vi "tcs shm issue Command stop Motion LV.vi"(8 "error in (no error)":errorcluster, 11 "command_stopMotion_Ctl":cluster{"stopMotion":u8}) -> (0 "error out":errorcluster, 2 "function return":i32, 3 "command_stopMotion_Ctl out":cluster{"stopMotion":u8})   [LabVIEW 2016, in "SALLV_tcs.lvlib"]
doc: "int tcs_shm_issueCommand_stopMotionLV(tcs_command_stopMotionLV *command_stopMotion_Ctl );"
uses:
  SALLV_tcs.lvlib
  SALLV_tcs.so
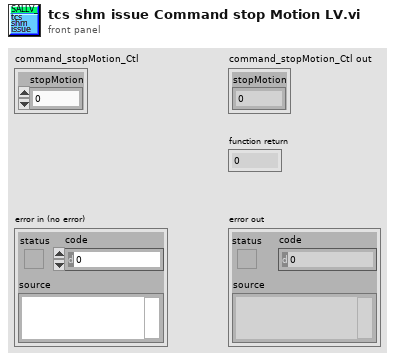
[diagram p1: front panel]
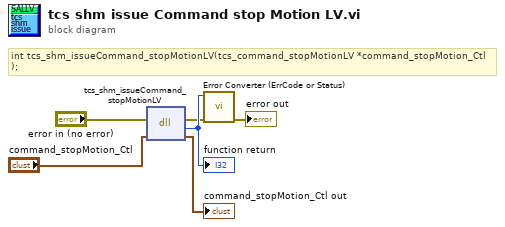
[diagram p0: block diagram]
diagram:
  # "int tcs_shm_issueCommand_stopMotionLV(tcs_command_stopMotionLV *command_stopMotion_Ctl );"
  n1 = dll-call lib="home/andres/Desktop/SALLV_tcs/SALLV_tcs.*" fn="tcs_shm_issueCommand_stopMotionLV"(error in="error in (no error)", "command_stopMotion_Ctl"="command_stopMotion_Ctl") -> (error out=w2:errorcluster, w6:i32, "command_stopMotion_Ctl"=→"command_stopMotion_Ctl out":cluster{"stopMotion":u8})  [unwired: 2 in, 1 out]
  "function return" <- w6
  n2 = call "Error Converter (ErrCode or Status).vi"("error in (no error)"=w2, "error code"=w6) -> ("error out"=→"error out":errorcluster)  [unwired: 9 in]
